vi "Initialize.vi"(0 "VISA resource name":refnum<visa-resource-name>, 5 "ID query (T:yes)":bool=TRUE, 9 "Reset (F:no)":bool, 11 "error in (no error)":errorcluster) -> (4 "VISA resource name out":refnum<visa-resource-name>, 15 "error out":errorcluster)   [LabVIEW 2012, in "Agilent 66XX Series.lvlib"]
doc: "This VI passes the addressing information in the instrument decriptor to the Instr Open VI and returns the instrument ID. You can optionally reset the instrument by setting the front panel reset control. You must run this VI before using any of the instrument driver VIs for this instrument."
uses:
  <instrlib>/Agilent 66XX Series/Agilent 66XX Series.lvlib
panel:
  # "© 2005 National Instruments.  ALL RIGHTS RESERVED."
  # "yes\nno"
  # "yes\nno"
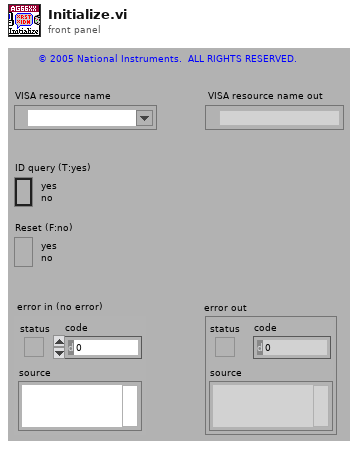
[diagram p1: front panel]
types:
  T1 = cluster{"status":bool, "code":i32, "VI name":string}
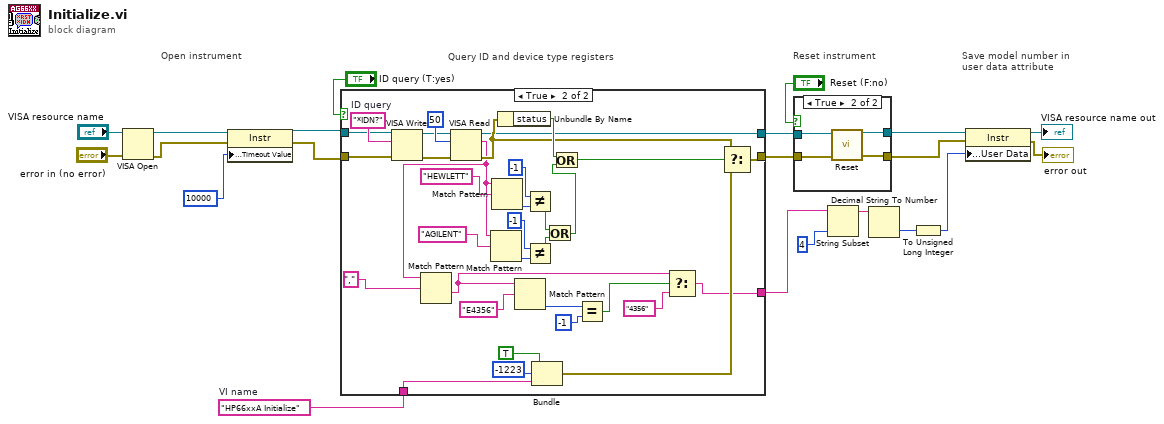
[diagram p0: block diagram]
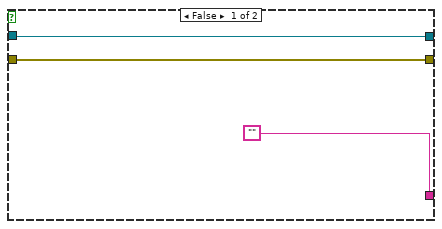
[diagram p3: hidden frame]
diagram:
  w9 = "HP66xxA Initialize"  # VI name
  # "Save model number in user data attribute"
  # "Query ID and device type registers"
  # "Reset instrument"
  # "Open instrument"
  n1 = VISA Open(error in (no error)="error in (no error)", VISA resource name="VISA resource name") -> (VISA resource name=w5:refnum<visa-resource-name>, error out=w4:errorcluster)  [unwired: 3 in]
  n2 = property class="Instr"(reference=w5, error in=w4, "General Settings:Timeout Value"=u32 10000 ("Tmo Value")) -> (reference out=w2:refnum<visa-resource-name>, error out=w3:errorcluster)
  n3 = case shown="True" "ID query (T:yes)" {
    tunnel: [w23 w55] -> w20
    tunnel: [w24 w40] -> w21
    tunnel: w9 -> [_ w53]
    tunnel: w2 -> [w24 w42]
    tunnel: w3 -> [w23 w45]
    tunnel: ["" w26] -> w16
    frame False {
    }
    frame True {
      w52 = "*IDN?"  # ID query
      n4 = VISA Write(VISA resource name=w42, write buffer=w52, error in (no error)=w45) -> (VISA resource name out=w41:refnum<visa-resource-name>, error out=w44:errorcluster)  [unwired: 1 out]
      n5 = VISA Read(VISA resource name=w41, byte count=u32 50, error in (no error)=w44) -> (VISA resource name out=w40:refnum<visa-resource-name>, read buffer=w32:string, error out=w43:errorcluster)  [unwired: 1 out]
      n6 = Match Pattern(string=w32, regular expression=",") -> (after substring=w27:string)  [unwired: 1 in, 3 out]
      n7 = Match Pattern(string=w32, regular expression="AGILENT") -> (offset past match=w38:i32)  [unwired: 1 in, 3 out]
      n8 = Match Pattern(string=w32, regular expression="HEWLETT") -> (offset past match=w50:i32)  [unwired: 1 in, 3 out]
      n9 = Unbundle By Name(w43) -> ("status"=w47:bool)
      n10 = Match Pattern(string=w27, regular expression="E4356" ("regular expression (\"\")")) -> (offset past match=w30:i32)  [unwired: 1 in, 3 out]
      n11 = Not Equal?(x=-1, y=w50) -> (x != y?=w35:bool)
      n12 = Not Equal?(x=-1, y=w38) -> (x != y?=w34:bool)
      n13 = Bundle(TRUE, -1223, "VI name"=w53) -> (w54:cluster{bool, i32, "VI name":string})  [unwired: 1 in]
      n14 = Or(x=w35, y=w34) -> (x .or. y?=w36:bool)
      n15 = Or(x=w47, y=w36) -> (x .or. y?=w46:bool)
      n16 = Equal?(x=w30, y=-1) -> (x = y?=w28:bool)
      n17 = Select(t=w27, s=w28, f="4356" ("replace string (\"\")")) -> (s? t:f=w26:string)
      n18 = Select(t=w43, s=w46, f=w54) -> (s? t:f=w55:T1)
    }
  }
  n19 = case shown="True" "Reset (F:no)" {
    tunnel: w20 -> [w59 w63]
    tunnel: [w59 w61] -> w7
    tunnel: w21 -> [w58 w62]
    tunnel: [w58 w60] -> w8
    frame False {
    }
    frame True {
      n20 = call <instrlib>:"Reset.vi"("VISA resource name"=w62, "error in (no error)"=w63) -> ("VISA resource name out"=w60:refnum<visa-resource-name>, "error out"=w61:errorcluster)  [unwired: 12 in]
    }
  }
  n21 = String Subset(string=w16, length (rest)=4) -> (substring=w14:string)  [unwired: 1 in]
  n22 = Decimal String To Number(string=w14) -> (number=w13:i32)  [unwired: 2 in, 1 out]
  n23 = To Unsigned Long Integer(number=w13) -> (unsigned 32bit integer=w10:u32)
  n24 = property class="Instr"(reference=w8, error in=w7, "General Settings:User Data"=w10) -> (reference out=→"VISA resource name out":refnum<visa-resource-name>, error out=→"error out":errorcluster)
